vi "Wait on Stop Sync.vi"(8 "error in":errorcluster, 11 "Stop Argument":T1={"Module ID"=-1, "Origin"="", "Exit via Stop Module Req?"=FALSE, "Wait for Module to stop?"=FALSE}) -> (0 "error out":errorcluster)   [LabVIEW 2024, in "Cloneable Subpanel.lvlib"]
doc: "Wait on the rendezvous that synchronizes the request to stop the module and the module stopping.\n\n_____\nBased on DQMH Dev Tools: Project Template 7.1.0.1499."
uses:
  Cloneable Subpanel.lvlib
  Stop Argument--cluster.ctl
  <vilib>/event_ctls.llb/usereventprio.ctl
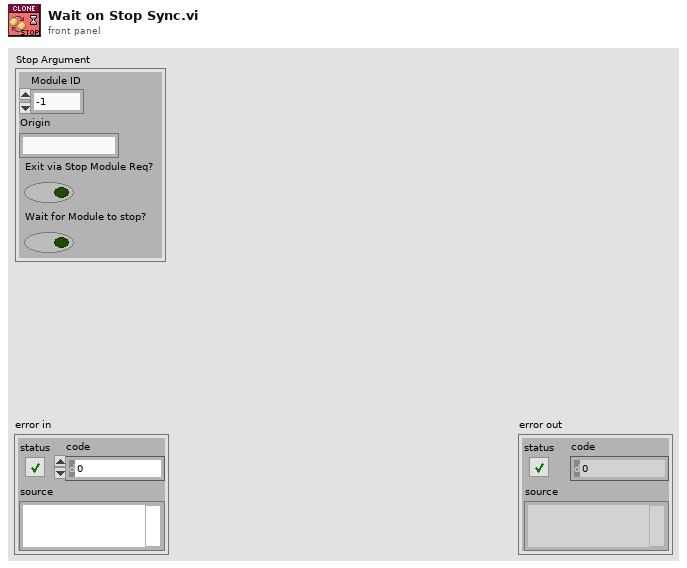
[diagram p1: front panel]
types:
  T1 = typedef "Cloneable Subpanel.lvlib/Stop Argument--cluster.ctl" = cluster{"Module ID":i32, "Origin":string, "Exit via Stop Module Req?":bool, "Wait for Module to stop?":bool}
  T2 = typedef "Cloneable Subpanel.lvlib/Request Events--cluster.ctl" = cluster{"Stop Module":refnum<user-event>, "Show Panel":refnum<user-event>, "Hide Panel":refnum<user-event>, "Show Diagram":refnum<user-event>, "Get Module Execution Status":refnum<user-event>}
  T3 = typedef "usereventprio.ctl" = enum32{"high priority", "normal priority"}
  T4 = typedef "Cloneable Subpanel.lvlib/Broadcast Events--cluster.ctl" = cluster{"Module Did Init":refnum<user-event>, "Status Updated":refnum<user-event>, "Error Reported":refnum<user-event>, "Module Did Stop":refnum<user-event>, "Update Module Execution Status":refnum<user-event>}
  T5 = typedef "Rendezvous RefNum" = refnum<k1>
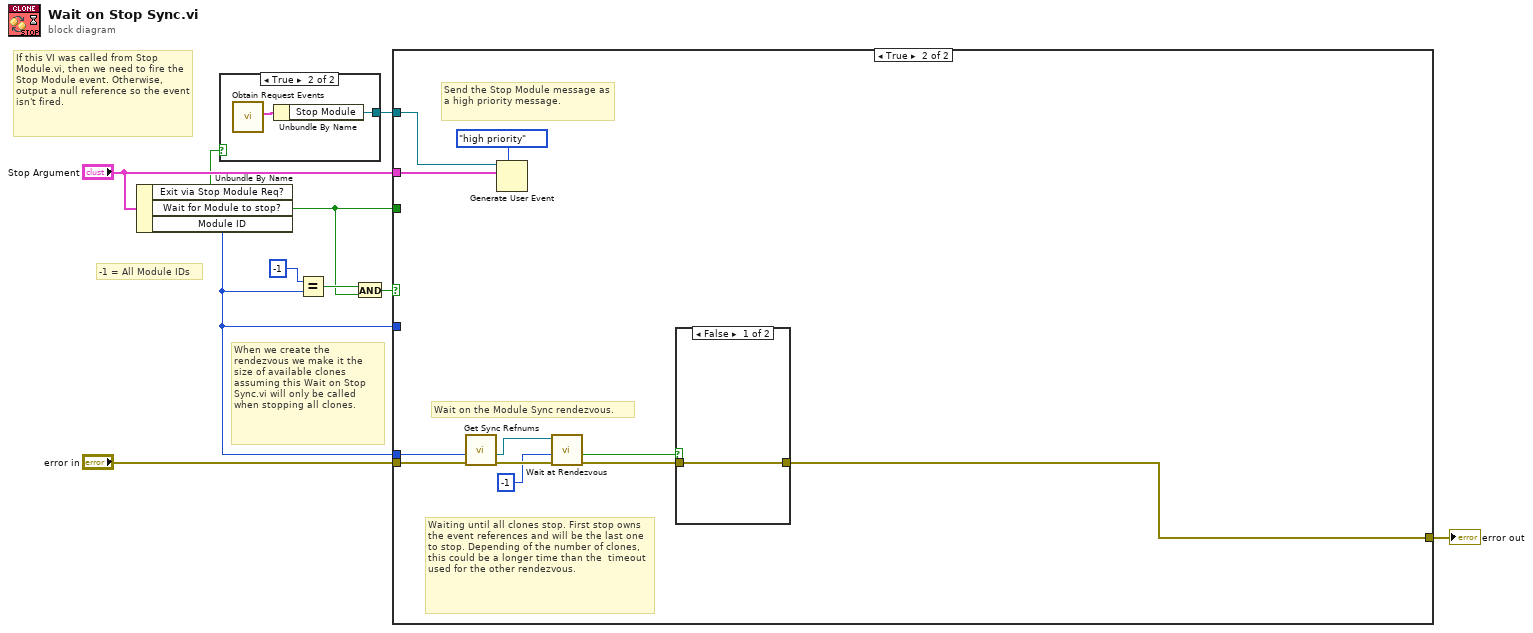
[diagram p0: block diagram]
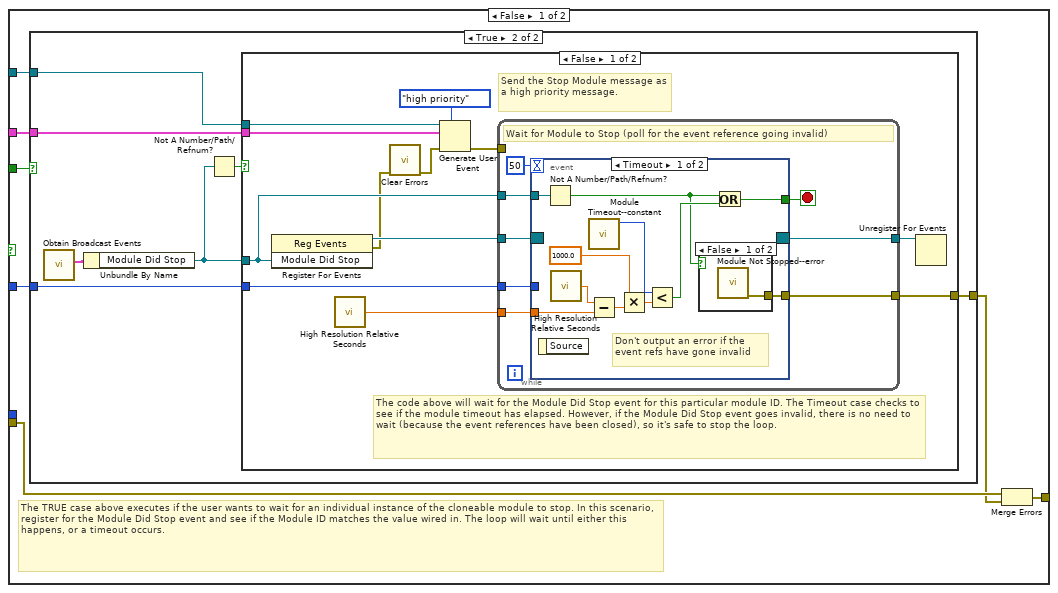
[diagram p3: hidden frame]
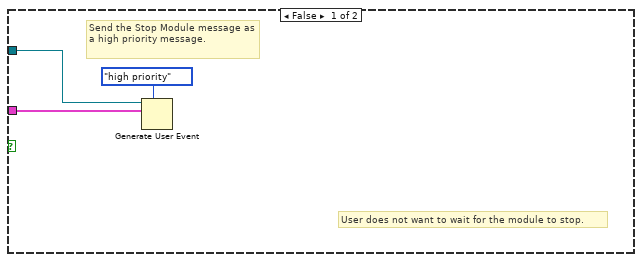
[diagram p4: hidden frame]
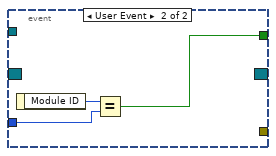
[diagram p6: hidden frame]
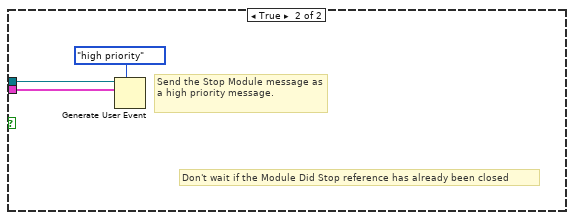
[diagram p7: hidden frame]
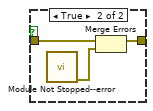
[diagram p8: hidden frame]
diagram:
  # "-1 = All Module IDs"
  # "If this VI was called from Stop Module.vi, then we need to fire the Stop Module event. Otherwise, output a null reference so the event isn't fired."
  # "When we create the rendezvous we make it the size of available clones assuming this Wait on Stop Sync.vi will only be called when stopping all clones."
  n1 = Unbundle By Name("Stop Argument") -> ("Exit via Stop Module Req?"=w2:bool, "Wait for Module to stop?"=w3:bool, "Module ID"=w1:i32)
  n2 = case shown="True" w2 {
    tunnel: [_ w11] -> w5
    frame False {
    }
    frame True {
      n3 = call "Obtain Request Events.vi"() -> ("Cloneable Subpanel Request Events"=w12:T2)  [unwired: 10 in, 1 out]
      n4 = Unbundle By Name(w12) -> ("Stop Module"=w11:refnum<user-event>)
    }
  }
  n5 = Equal? ("When we create the rendezvous we\nmake it the size of available clones assuming this Wait on Stop Sync.vi will only be called when stopping all clones.")(x=-1, y=w1) -> (x = y?=w7:bool)
  n6 = And(x=w7, y=w3) -> (x .and. y?=w6:bool)
  n7 = case shown="True" w6 {
    tunnel: "error in" -> [w19 w78]
    tunnel: [w18 w75] -> w9
    tunnel: w1 -> [_ w72]
    tunnel: w3 -> [w16 _]
    tunnel: w1 -> [w15 _]
    tunnel: w5 -> [w14 w69]
    tunnel: "Stop Argument" -> [w13 w70]
    frame False {
      # "The TRUE case above executes if the user wants to wait for an individual instance of the cloneable module to stop. In this scenario, register for the Module Did Stop event and see if the Module ID matches the value wired in. The loop will wait until either this happens, or a timeout occurs."
      n8 = case shown="True" w16 {
        tunnel: w15 -> [_ w27]
        tunnel: [_ w29] -> w17
        tunnel: w14 -> [w20 w23]
        tunnel: w13 -> [w21 w24]
        frame False {
          # "Send the Stop Module message as a high priority message."
          # "User does not want to wait for the module to stop."
          n9 = Generate User Event(priority (normal)=usereventprio."high priority", user event=w20, event data cluster=w21) -> ()  [unwired: 1 in, 2 out]
        }
        frame True {
          n10 = call "Obtain Broadcast Events.vi"() -> ("Cloneable Subpanel Broadcast Events"=w28:T4)  [unwired: 10 in, 1 out]
          n11 = Unbundle By Name(w28) -> ("Module Did Stop"=w26:refnum<user-event>)
          n12 = Not A Number/Path/Refnum?(number/path/refnum=w26) -> (NaN/Path/Refnum?=w25:bool)
          n13 = case shown="False" w25 {
            tunnel: w27 -> [w39 _]
            tunnel: [w41 _] -> w29
            tunnel: w26 -> [w37 _]
            tunnel: w24 -> [w34 w66]
            tunnel: w23 -> [w33 w65]
            frame False {
              # "Send the Stop Module message as a high priority message."
              # "The code above will wait for the Module Did Stop event for this particular module ID. The Timeout case checks to see if the module timeout has elapsed. However, if the Module Did Stop event goes invalid, there is no need to wait (because the event references have been closed), so it's safe to stop the loop."
              n14 = register-events(w37) -> (reference out=w40:refnum<event-registration>, error out=w32:errorcluster)  [unwired: 2 in]
              n15 = call <vilib>:"High Resolution Relative Seconds.vi"() -> ("relative seconds"=w36:dbl)
              n16 = call <vilib>:"Clear Errors.vi"("error in (no error)"=w32) -> ("error out"=w31:errorcluster)  [unwired: 5 in, 1 out]
              n17 = Generate User Event(priority (normal)=usereventprio."high priority", user event=w33, event data cluster=w34, error in=w31) -> (error out=w30:errorcluster)  [unwired: 1 out]
              n18 = while {
                tunnel: w40 -> [w48]
                tunnel: w39 -> [w46]
                tunnel: [w49] -> w41
                tunnel: [w45] -> w38
                tunnel: w37 -> [w43]
                tunnel: w36 -> [w42]
                tunnel: w30 -> [_]
                stop <- w47 stop-if-true
                # "Wait for Module to Stop (poll for the event reference going invalid)"
                n19 = event shown="[0] Timeout" {
                  selector: w48 -> [_ _]
                  dyn-events: [_ _] -> w45
                  timeout: 50 -> [_ _]
                  tunnel: [w58 w62] -> w47
                  tunnel: w46 -> [_ w63]
                  tunnel: [w60 _] -> w49
                  tunnel: w43 -> [w59 _]
                  tunnel: w42 -> [w57 _]
                  event Timeout {
                    # "Don't output an error if the event refs have gone invalid"
                    n20 = event-data() -> ()  [unwired: 1 in, 1 out]
                    n21 = Not A Number/Path/Refnum?(number/path/refnum=w59) -> (NaN/Path/Refnum?=w50:bool)
                    n22 = call <vilib>:"High Resolution Relative Seconds.vi"() -> ("relative seconds"=w56:dbl)
                    n23 = call "Module Timeout--constant.vi"() -> ("Module Timeout"=w52:i32)  [unwired: 11 in]
                    n24 = Subtract(x=w56, y=w57) -> (x-y=w55:dbl)
                    n25 = Multiply(x=1000.0, y=w55) -> (x*y=w53:dbl)
                    n26 = Less?(x=w52, y=w53) -> (x < y?=w51:bool)
                    n27 = case shown="False" w50 {
                      tunnel: [w61 _] -> w60
                      frame False {
                        n28 = call "Module Not Stopped--error.vi"() -> ("error out"=w61:errorcluster)  [unwired: 11 in]
                      }
                      frame True {
                      }
                    }
                    n29 = Or(x=w50, y=w51) -> (x .or. y?=w58:bool)
                  }
                  event User Event {
                    n30 = event-data() -> ("Module ID"=w64:i32)  [unwired: 1 in]
                    n31 = Equal?(x=w64, y=w63) -> (x = y?=w62:bool)
                  }
                }
              }
              n32 = Unregister For Events(event registration refnum=w38) -> ()  [unwired: 1 in, 1 out]
            }
            frame True {
              # "Send the Stop Module message as a high priority message."
              # "Don't wait if the Module Did Stop reference has already been closed"
              n33 = Generate User Event(priority (normal)=usereventprio."high priority", user event=w65, event data cluster=w66) -> ()  [unwired: 1 in, 2 out]
            }
          }
        }
      }
      n34 = Merge Errors(w19, w17) -> (w18:errorcluster)
    }
    frame True {
      # "Waiting until all clones stop. First stop owns the event references and will be the last one to stop. Depending of the number of clones, this could be a longer time than the  timeout used for the other rendezvous."
      # "Send the Stop Module message as a high priority message."
      # "Wait on the Module Sync rendezvous."
      n35 = call "Get Sync Refnums.vi"("error in"=w78, "Module ID"=w72) -> ("error out"=w77:errorcluster, "Stop Sync"=w71:T5)  [unwired: 6 in, 2 out]
      n36 = Generate User Event(priority (normal)=usereventprio."high priority", user event=w69, event data cluster=w70) -> ()  [unwired: 1 in, 2 out]
      n37 = call <vilib>:"Wait at Rendezvous.vi"("error in (no error)"=w77, "ms timeout (-1)"=-1, "rendezvous"=w71) -> ("error out"=w76:errorcluster, "timed out"=w73:bool)  [unwired: 2 in, 1 out]
      n38 = case shown="False" w73 {
        tunnel: w76 -> [w79 w82]
        tunnel: [w79 w81] -> w75
        frame False {
        }
        frame True {
          n39 = call "Module Not Stopped--error.vi"() -> ("error out"=w80:errorcluster)  [unwired: 11 in]
          n40 = Merge Errors(w82, w80) -> (w81:errorcluster)
        }
      }
    }
  }
  "error out" <- w9
